vi "Function.vi"(8 "error in (no error)":errorcluster, 9 "Numeric B":T1, 10 "Numeric A":T1, 11 "Two Terminal in":refnum<class "AbsFunc_Two Term_U16.lvclass">) -> (0 "error out":errorcluster, 2 "Result":T1, 3 "Two Terminal out":refnum<class "AbsFunc_Two Term_U16.lvclass">)   [LabVIEW 2021, in "AbsFunc_Two Term_U16.lvclass"]
uses:
  AbsFunc_Two Term_U16.lvclass
  Support/Data Type.ctl
  AbsFunc_Two Term_U16.lvclass/AbsFunc_Two Term_U16.ctl
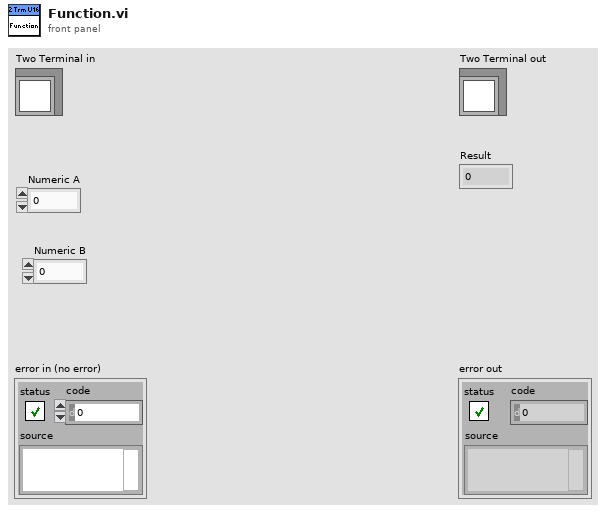
[diagram p1: front panel]
types:
  T1 = typedef "AbsFunc_Two Term_U16.lvclass/Data Type.ctl" = u16
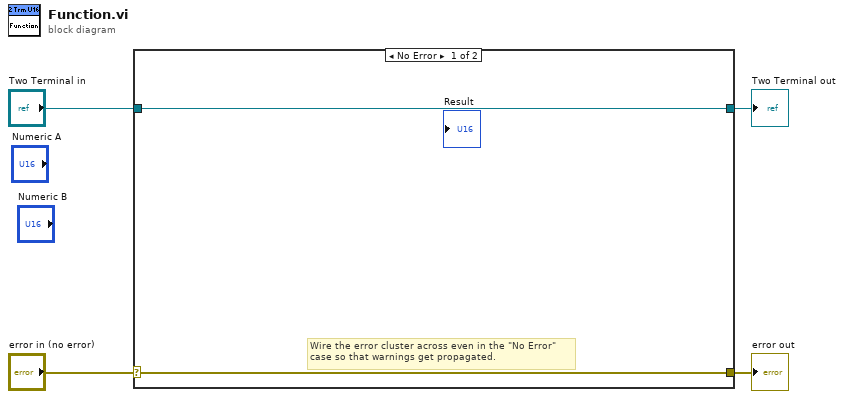
[diagram p0: block diagram]
diagram:
  n1 = case shown="No Error" "error in (no error)" {
    selector: "error in (no error)" -> [w5 w8]
    tunnel: [w5 w8] -> w3
    tunnel: [w6 w7] -> w1
    tunnel: "Two Terminal in" -> [w6 w7]
    frame No Error {
      # "Wire the error cluster across even in the \"No Error\"\ncase so that warnings get propagated."
    }
    frame Error {
    }
  }
  "error out" <- w3
  "Two Terminal out" <- w1
